vi "Handle Data.vi"(8 "error in (no error)":errorcluster, 10 "Data":dbl, 11 "CoolApp in":refnum<class "CoolApp.lvclass">) -> (0 "error out":errorcluster, 3 "CoolApp out":refnum<class "CoolApp.lvclass">)   [LabVIEW 2020, in "LAF2024Q2.lvlib" / "CoolApp.lvclass"]
uses:
  CoolApp.lvclass
  Nested.ctl
  CoolApp.lvclass/CoolApp.ctl
  DataHandler Messages/Handle Data Msg/Handle Data Msg.lvclass/Handle Data Msg.ctl
  <vilib>/ActorFramework/Message Enqueuer/Message Enqueuer.lvclass/Message Enqueuer.ctl
  <vilib>/ActorFramework/Message Enqueuer/Enqueue.vi
  DataHandler Messages/Handle Data Msg/Handle Data Msg.lvclass
  C:/Program Files (x86)/National Instruments/LabVIEW 2020/vi.lib/ActorFramework/Message/Message.lvclass
  <vilib>/ActorFramework/Message Priority Queue/Priority Enqueue.vi
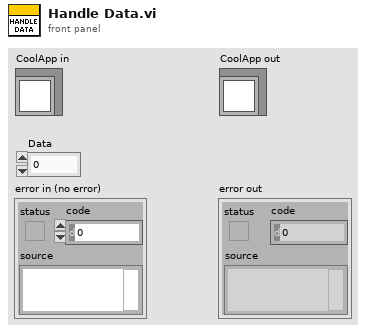
[diagram p1: front panel]
types:
  T1 = typedef "LAF2024Q2.lvlib/CoolApp.lvclass/Nested.ctl" = enum16{"DAQ", "Chart"}
  T2 = map{T1, refnum<class "Message Enqueuer.lvclass">}
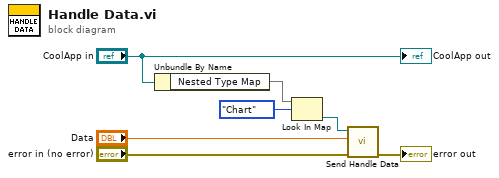
[diagram p0: block diagram]
diagram:
  n1 = Unbundle By Name("CoolApp in") -> ("Nested Type Map"=w6:T2)
  n2 = Look In Map(map=w6, key=Nested."Chart") -> (value=w3:refnum<class "Message Enqueuer.lvclass">)  [unwired: 1 in, 1 out]
  n3 = call "Send Handle Data.vi"("error in (no error)"="error in (no error)", "Data"="Data", "Message Enqueuer"=w3) -> ("error out"=→"error out":errorcluster)  [unwired: 7 in, 1 out]
  "CoolApp out" <- "CoolApp in"
